vi "High Precision Timer.vi"() -> (0 "?":ext format="%.9f")   [LabVIEW 2011]
doc: "Wiebe Walstra\nwiebe.walstra@carya.nl\n\nCarya Automatisering\nwww.carya.nl\n\nFebruari 2004"
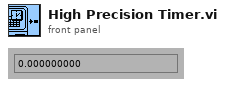
[diagram p1: front panel]
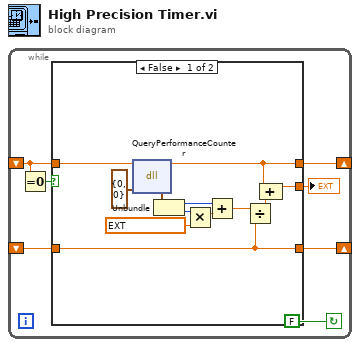
[diagram p0: block diagram]
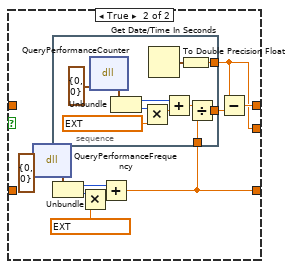
[diagram p2: hidden frame]
diagram:
  n1 = while {
    shift-left: _ -> [w5]
    shift-right: [w6] -> _
    shift-left: _ -> [w3]
    shift-right: [w7] -> _
    stop <- FALSE continue-if-true
    n2 = Equal To 0?(x=w3) -> (x = 0?=w2:bool)
    n3 = case shown="False" w2 {
      tunnel: [w9 w20] -> w7
      tunnel: [w11 w22] -> w6
      tunnel: w5 -> [w11 _]
      tunnel: w3 -> [w9 _]
      tunnel: [w10 w19] -> w4
      frame False {
        n4 = dll-call lib="kernel32" fn="QueryPerformanceCounter"(cluster{u32, u32} {0, 0}) -> (w13:cluster{u32, u32})  [unwired: 3 in, 3 out]
        n5 = Unbundle(w13) -> (w14:u32, w17:u32)
        n6 = Multiply(x=w17, y=ext 4294967295.0) -> (x*y=w15:ext)
        n7 = Add(x=w14, y=w15) -> (x+y=w12:ext)
        n8 = Divide(x=w12, y=w11) -> (x/y=w8:ext)
        n9 = Compound Arithmetic op=ADD(w9, w8) -> (w10:ext)
      }
      frame True {
        n10 = dll-call lib="kernel32" fn="QueryPerformanceFrequency"(cluster{u32, u32} {0, 0}) -> (w23:cluster{u32, u32})  [unwired: 3 in, 3 out]
        n11 = Unbundle(w23) -> (w24:u32, w27:u32)
        n12 = Multiply(x=w27, y=ext 4294967295.0) -> (x*y=w25:ext)
        n13 = Add(x=w24, y=w25) -> (x+y=w22:ext)
        n14 = stacked-sequence {
          tunnel: w22 -> [w32]
          tunnel: [w31] -> w19
          tunnel: [w30] -> w21
          frame #0 {
            n15 = dll-call lib="kernel32" fn="QueryPerformanceCounter"(cluster{u32, u32} {0, 0}) -> (w34:cluster{u32, u32})  [unwired: 3 in, 3 out]
            n16 = Unbundle(w34) -> (w35:u32, w38:u32)
            n17 = Multiply(x=w38, y=ext 4294967295.0) -> (x*y=w36:ext)
            n18 = Get Date/Time In Seconds() -> (seconds since 1Jan1904=w29:timestamp)
            n19 = Add(x=w35, y=w36) -> (x+y=w33:ext)
            n20 = To Double Precision Float(number=w29) -> (double precision float=w31:dbl)
            n21 = Divide(x=w33, y=w32) -> (x/y=w30:ext)
          }
        }
        n22 = Subtract(x=w19, y=w21) -> (x-y=w20:ext)
      }
    }
    "?" <- w4
  }
